vi "tip_date_03.vi"() -> ()   [LabVIEW 2010]
panel:
  out "Waveform Chart":cluster{"Knob":dbl, "Knob 2":dbl}(graph)
  in  "Knob 2":dbl(knob) scale=0.0..100.0
  in  "Knob":dbl(knob) scale=0.0..100.0
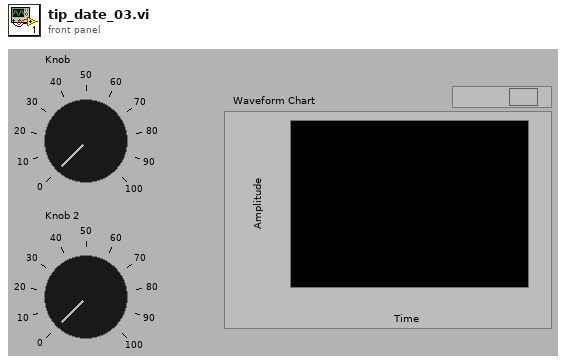
[diagram p1: front panel]
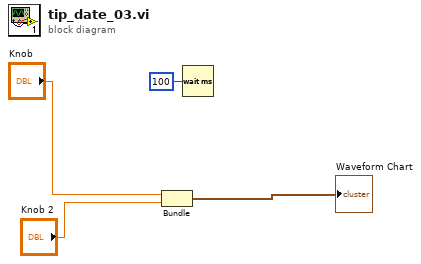
[diagram p0: block diagram]
diagram:
  n1 = Bundle("Knob"="Knob", "Knob 2"="Knob 2") -> (→"Waveform Chart":cluster{"Knob":dbl, "Knob 2":dbl})  [unwired: 1 in]
  n2 = Wait (ms)(milliseconds to wait=u32 100) -> ()  [unwired: 1 out]
